vi "mod_Rayleigh Fading (Gans).vi"(0 "profile length (samples)":i32=1000, 5 "sampling frequency (Hz)":dbl=1.0 format="%.2f", 7 "doppler spread (Hz)":dbl=0.01 format="%.2p", 9 "seed in (0xFFFFFFFF)":i32=-1 format="%.0x", 11 "error in (no error)":errorcluster, 12 "fading variance":dbl=1.0 format="%.2f", 13 "reset? (T)":bool=TRUE) -> (4 "rayleigh fading profile":cdb[](array[numeric]) format="%.2f", 10 "seed out":i32 format="%.0x", 15 "error out":errorcluster)   [LabVIEW 2020, in "niDMT.lvlib"]
doc: "The Rayleigh fading channel is generated based on Clarke and Gans Model using the Doppler filter with U-shaped power spectral density. \n \n\n Inputs:\n 1) Doppler spread (Hz) \n - range : double precision (default:20)\n - an example : a running vehicle with 65mph (104km/h), the carrier frequency of 900MHz\n The speed of the vehicle = 65*1.6*1000/3600 = 28.89m/s\n Doppler frequency = (900MHz)*(28.89m/s)/(300*10^6m/s) = 86.67 Hz\n 2) Fading variance : the variance of the fading channel output\n - range : double precision (default:2)\n 3) Input waveform : Input signal samples\n - some default values were set.\n (dt:0.00025, the number of samples:4000)\n 4) seed in (0xFFFFFFFF)\n 5) Error in\n\n Outputs:\n 1) Rayleigh fading profile : the complex fading channel output\n 2) Error out"
uses:
  <vilib>/addons/Modulation/niDMT.lvlib
  <vilib>/addons/Modulation/niAMT.lvlib
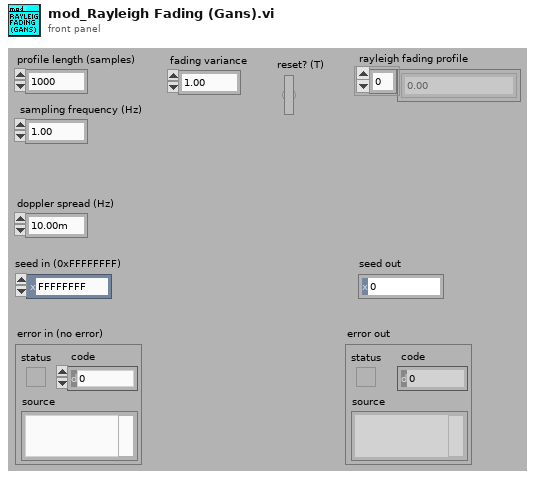
[diagram p1: front panel]
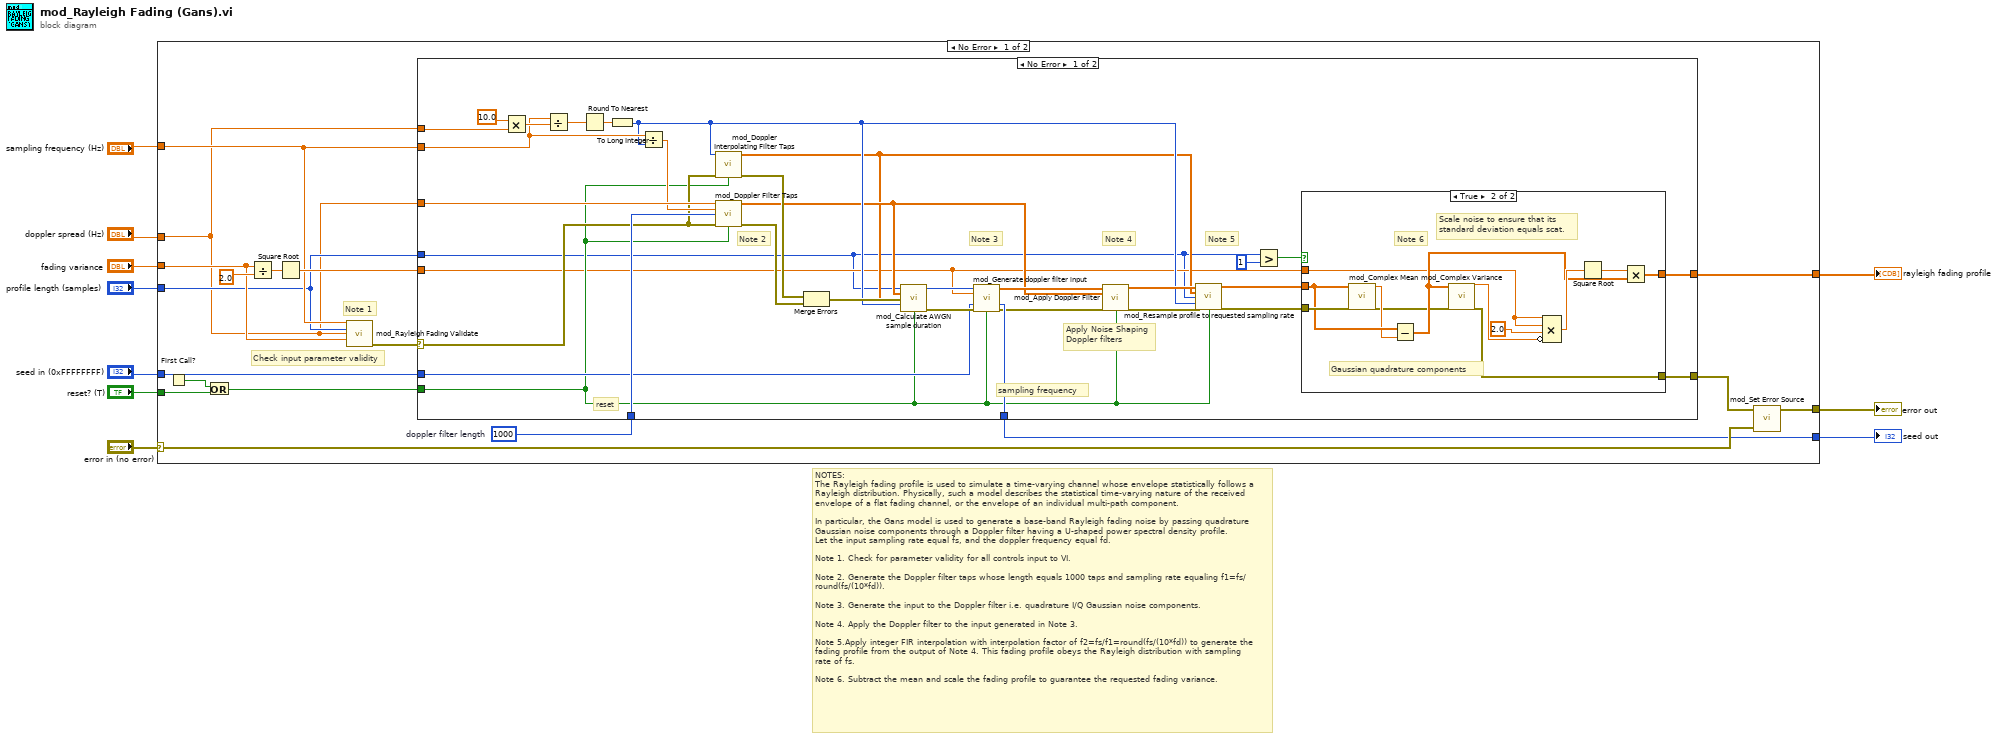
[diagram p0: block diagram]
diagram:
  # "NOTES:\nThe Rayleigh fading profile is used to simulate a time-varying channel whose envelope statistically follows a Rayleigh distribution. Physically, such a model describes the statistical time-varying nature of the received envelope of a flat fading channel, or the envelope of an individual multi-path component.\n\t\t  \nIn particular, the Gans model is used to generate a base-band Rayleigh fading noise by passing quadrature Gaussian noise components through a Doppler filter having a U-shaped power spectral density profile. \nLet the input sampling rate equal fs, and the doppler frequency equal fd.\n\nNote 1. Check for parameter validity for all controls input to VI.\n\nNote 2. Generate the Doppler filter taps whose length equals 1000 taps and sampling rate equaling f1=fs/round(fs/(10*fd)).\n\nNote 3. Generate the input to the Doppler filter i.e. quadrature I/Q Gaussian noise components.\n\nNote 4. Apply the Doppler filter to the input generated in Note 3.\n\nNote 5.Apply integer FIR interpolation with interpolation factor of f2=fs/f1=round(fs/(10*fd)) to generate the fading profile from the output of Note 4. This fading profile obeys the Rayleigh distribution with sampling\nrate of fs. \n\nNote 6. Subtract the mean and scale the fading profile to guarantee the requested fading variance."
  n1 = case shown="No Error" "error in (no error)" {
    selector: "error in (no error)" -> [w26 w77]
    tunnel: [w27 w77] -> w10
    tunnel: [w28 _] -> w8
    tunnel: "sampling frequency (Hz)" -> [w18 _]
    tunnel: "doppler spread (Hz)" -> [w13 _]
    tunnel: "fading variance" -> [w17 _]
    tunnel: "profile length (samples)" -> [w16 _]
    tunnel: "seed in (0xFFFFFFFF)" -> [w15 _]
    tunnel: "reset? (T)" -> [w14 _]
    tunnel: [w12 _] -> w1
    frame No Error {
      w11 = 1000  # doppler filter length
      # "Note 1"
      # "Check input parameter validity"
      n2 = First Call?() -> (First Call?: T/F=w22:bool)
      n3 = Or(x=w22, y=w14) -> (x .or. y?=w19:bool)
      n4 = Divide(x=w17, y=2.0) -> (x/y=w21:dbl)
      n5 = Square Root(x=w21) -> (sqrt(x)=w23:dbl)
      n6 = call <vilib>:"mod_Rayleigh Fading Validate.vi"("sampling frequency"=w18, "profile length (samples)"=w16, "doppler spread (Hz)"=w13, "fading variance"=w17) -> ("error out"=w24:errorcluster)  [unwired: 11 out]
      n7 = case shown="No Error" w24 {
        selector: w24 -> [w45 w76]
        tunnel: [w61 _] -> w28
        tunnel: w13 -> [w59 _]
        tunnel: w16 -> [w31 _]
        tunnel: w23 -> [w32 _]
        tunnel: [w60 w76] -> w25
        tunnel: w19 -> [w36 _]
        tunnel: w15 -> [w37 _]
        tunnel: w18 -> [w47 _]
        tunnel: w13 -> [w49 _]
        tunnel: [w54 _] -> w12
        tunnel: w11 -> [w51 _]
        frame No Error {
          # "Note 5"
          # "Note 4"
          # "Note 3"
          # "Note 2"
          # "reset"
          # "sampling frequency"
          # "Apply Noise Shaping Doppler filters"
          n8 = Multiply(x=10.0, y=w49) -> (x*y=w48:dbl)
          n9 = Divide(x=w47, y=w48) -> (x/y=w53:dbl)
          n10 = Round To Nearest(number=w53) -> (nearest integer value=w46:dbl)
          n11 = To Long Integer(number=w46) -> (32bit integer=w35:i32)
          n12 = Divide(x=w47, y=w35) -> (x/y=w52:dbl)
          n13 = call <vilib>:"mod_Doppler Interpolating Filter Taps.vi"("interpolation factor"=w35, "error in (no error)"=w45, "reset? (T)"=w36) -> ("interpolating filter taps"=w33:dbl[], "error out"=w42:errorcluster)  [unwired: 11 out]
          n14 = call <vilib>:"mod_Doppler Filter Taps.vi"("doppler spread (hz)"=w59, "fs"=w52, "doppler filter length"=w51, "error in (no error)"=w45, "reset? (T)"=w36) -> ("doppler filter taps"=w34:dbl[], "error out"=w41:errorcluster)  [unwired: 1 in, 8 out]
          n15 = Merge Errors(w42, w41) -> (w40:errorcluster)
          n16 = call <vilib>:"mod_Calculate AWGN sample duration.vi"("profile length (samples)"=w31, "doppler filter taps"=w34, "interpolating filter taps"=w33, "interpolation factor"=w35, "error in (no error)"=w40, "reset? (T)"=w36) -> ("AWGN samples"=w39:i32, "error out"=w38:errorcluster)  [unwired: 8 out]
          n17 = call <vilib>:"mod_Generate doppler filter input.vi"("profile length (samples)"=w39, "standard deviation"=w32, "seed in (0xFFFFFFFF)"=w37, "error in (no error)"=w38, "reset? (T)"=w36) -> ("doppler filter input"=w58:cdb[], "seed out"=w54:i32, "error out"=w44:errorcluster)  [unwired: 3 in, 5 out]
          n18 = call <vilib>:"mod_Apply Doppler Filter.vi"("input samples"=w58, "doppler filter taps"=w34, "error in (no error)"=w44, "reset (T)"=w36) -> ("filtered output"=w57:cdb[], "error out"=w43:errorcluster)  [unwired: 2 in, 8 out]
          n19 = call <vilib>:"mod_Resample profile to requested sampling rate.vi"("doppler filter output"=w57, "interpolating filter"=w33, "profile length (samples)"=w31, "interpolation factor"=w35, "error in (no error)"=w43, "reset? (T)"=w36) -> ("fading profile"=w55:cdb[], "error out"=w56:errorcluster)  [unwired: 8 out]
          n20 = Greater?(x=w31, y=1) -> (0:w29:bool)
          n21 = case shown="True" w29 {
            tunnel: [w63 w74] -> w61
            tunnel: [w62 w73] -> w60
            tunnel: w56 -> [w62 w72]
            tunnel: w55 -> [w63 w71]
            tunnel: w32 -> [_ w64]
            frame False {
              # "If requested fading profile duration=1 sample, it is meaningless\nto subtract mean and scale for variance."
            }
            frame True {
              # "Note 6"
              # "Scale noise to ensure that its\nstandard deviation equals scat."
              # "Gaussian quadrature components"
              n22 = call <vilib>:"mod_Complex Mean.vi"("Signal In"=w71, "error in (no error)"=w72) -> ("Mean"=w70:cdb, "error out"=w68:errorcluster)  [unwired: 12 out]
              n23 = Subtract(x=w71, y=w70) -> (x-y=w69:cdb[])
              n24 = call <vilib>:"mod_Complex Variance.vi"("Signal In"=w69, "error in (no error)"=w68) -> ("Variance"=w67:dbl, "error out"=w73:errorcluster)  [unwired: 12 out]
              n25 = Compound Arithmetic op=MULTIPLY(w64, w64, 2.0 ("value"), invert w67) -> (w75:dbl)
              n26 = Square Root(x=w75) -> (sqrt(x)=w65:dbl)
              n27 = Multiply(x=w65, y=w69) -> (x*y=w74:cdb[])
            }
          }
        }
        frame Error {
        }
      }
      n28 = call <vilib>:"mod_Set Error Source.vi"("initial error in (no error)"=w26, "final error in (no error)"=w25) -> ("error out"=w27:errorcluster)  [unwired: 1 in, 2 out]
    }
    frame Error {
    }
  }
  "error out" <- w10
  "rayleigh fading profile" <- w8
  "seed out" <- w1
